vi "Test_getEvent_summaryState.vi"(8 "error in (no error)":errorcluster, 11 "logevent_summaryState_Ctl":T1) -> (0 "error out":errorcluster, 2 "function return":i32, 3 "logevent_summaryState_Ctl out":T1)   [LabVIEW 2016, in "SALLV_Test.lvlib"]
doc: "int Test_shm_getEvent_summaryStateLV(Test_logevent_summaryStateLV *logevent_summaryState_Ctl );"
uses:
  SALLV_Test.lvlib
  DataTypes/logevent_summaryState.ctl
  SALLV_Test.so
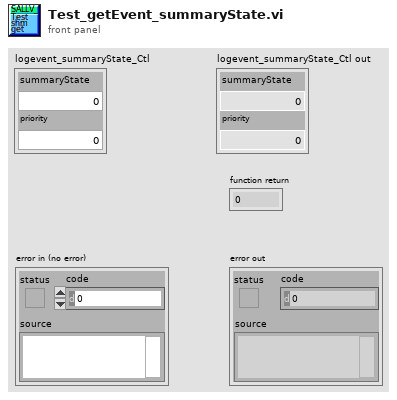
[diagram p1: front panel]
types:
  T1 = typedef "SALLV_Test.lvlib/logevent_summaryState.ctl" = cluster{"summaryState":i32, "priority":i32}
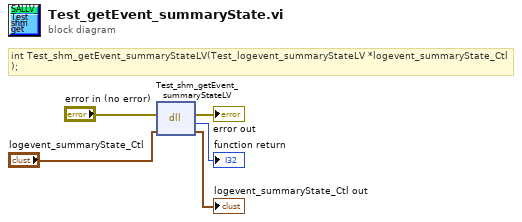
[diagram p0: block diagram]
diagram:
  # "int Test_shm_getEvent_summaryStateLV(Test_logevent_summaryStateLV *logevent_summaryState_Ctl );"
  n1 = dll-call lib="home/ccontaxis/Code/SALLV_Test/SALLV_Test.*" fn="Test_shm_getEvent_summaryStateLV"(error in="error in (no error)", "logevent_summaryState_Ctl"="logevent_summaryState_Ctl") -> (error out=→"error out":errorcluster, →"function return":i32, "logevent_summaryState_Ctl"=→"logevent_summaryState_Ctl out":T1)  [unwired: 2 in, 1 out]
